vi "Host - REF - MAIN.vi"() -> ()   [LabVIEW 2015]
doc: "This VI initializes de FPGA VI and then configures the DMA FIFO to read streaming data from the FPGA. Once the data is read from the FIFO it is de-interleaved and organized by channels."
uses:
  <vilib>/LabVIEW Targets/FPGA/cRIO/shared/nicrio_ModuleControls/nicrio_cRIO-9234_DataRatesRing2.ctl
  <vilib>/userdefined/High Color/nirio_resource_hc.ctl
  <vilib>/FPGAPlugInAG/cRIO-9112/niLvFpga_Open_cRIO-9112.vi
  <vilib>/rvi/interface/common/dynamic/niFpgaDynamicAddResources.vi
  <vilib>/FPGAPlugInAG/Dynamic/niLvFpga_Reset_Dynamic.vi
  <vilib>/FPGAPlugInAG/Dynamic/niLvFpga_Run_Dynamic.vi
  <vilib>/rvi/errors/niLvFpgaAdjustHostInterfaceError.vi
  <vilib>/rvi/interface/common/niFpgaWaitOnOcc.vi
  <vilib>/RVI Host/nirviSupport.llb/nirviErrorClusterFromErrorCode.vi
  <vilib>/FPGAPlugInAG/Dynamic/niLvFpga_Close_Dynamic.vi
  <vilib>/rvi/interface/nirviOpenFPGA/nirviOpenFPGA.xnode
  FPGA Bitfiles/REF1 - 2 Modules/AmbientSynchrono_FPGATarget2_Target-REF1-mod6-7.lvbitx
  <vilib>/rvi/interface/nirviMethod/nirviMethod.xnode
  <vilib>/rvi/interface/nirviReadWriteControl/nirviReadWriteControl.xnode
  <vilib>/rvi/interface/nirviCloseFPGA/nirviCloseFPGA.xnode
  <vilib>/rvi/interface/Simulation/niFpgaSimulationCallBeginRW.vi
  <vilib>/rvi/errors/niLvFpgaMergeErrorWithErrorCode.vi
  <vilib>/FPGAPlugInAG/Dynamic/niLvFpga_ReadFifo_Dynamic.vi
  NiFpgaLv.dll
  <vilib>/FPGAPlugInAG/Dynamic/niLvFpga_ConfigureFifo_Dynamic.vi
  <vilib>/FPGAPlugInAG/Dynamic/niLvFpga_StartFifo_Dynamic.vi
  <vilib>/rvi/interface/nirviMethod/StockFPGA_InlinedMethodWaitForSingleIRQ.vi
  <vilib>/FPGAPlugInAG/Dynamic/niLvFpga_WaitOnIrq_Dynamic.vi
  <vilib>/FPGAPlugInAG/Dynamic/niLvFpga_AcknowledgeIrq_Dynamic.vi
  <vilib>/FPGAPlugInAG/Dynamic/niLvFpga_StopFifo_Dynamic.vi
panel:
  out "Current Free Space (Mb)":dbl
  out "Low on Free Disk Space":bool
  in  "Save Type":u16(ring) items=["USB", "cRIO"]
  out "?":dbl[][](graph)
  out "Bin Header Check":i32
  in  "Filename":string
  out "UTC offset valid":bool
  out "UTC Offset":i8
  out "Satellites":u8
  out "Antenna Status":T1(ring)
  out "Offset From Time Reference":i32
  out "FPGA Timekeeper locked":bool
  out "GPS status":T2(ring)
  in  "Resource Name":T3 caption="RIO Device"
  out "error out":errorcluster
  out "Elements Remaining":u32
  in  "Stream to Disk":bool
  out "Module Underflow":bool
  out "DMA FIFO Full":bool
  in  "stop":bool
  in  "Data Rate":T4=31 items=["51.200 kS/s (NI 9234)"=1, "25.600 kS/s (NI 9234)"=2, "17.067 kS/s (NI 9234)"=3, "12.800 kS/s (NI 9234)"=4, "10.240 kS/s (NI 9234)"=5, "8.533 kS/s (NI 9234)"=6, "7.314 kS/s (NI 9234)"=7, "6.400 kS/s (NI 9234)"=8, "5.689 kS/s (NI 9234)"=9, "5.120 kS/s (NI 9234)"=10, "4.654 kS/s (NI 9234)"=11, "4.267 kS/s (NI 9234)"=12, "3.938 kS/s (NI 9234)"=13, "3.657 kS/s (NI 9234)"=14, "3.413 kS/s (NI 9234)"=15, "3.200 kS/s (NI 9234)"=16, "3.012 kS/s (NI 9234)"=17, "2.845 kS/s (NI 9234)"=18, "2.695 kS/s (NI 9234)"=19, "2.560 kS/s (NI 9234)"=20, "2.438 kS/s (NI 9234)"=21, "2.328 kS/s (NI 9234)"=22, "2.226 kS/s (NI 9234)"=23, "2.133 kS/s (NI 9234)"=24, "2.048 kS/s (NI 9234)"=25, "1.969 kS/s (NI 9234)"=26, "1.896 kS/s (NI 9234)"=27, "1.829 kS/s (NI 9234)"=28, "1.765 kS/s (NI 9234)"=29, "1.707 kS/s (NI 9234)"=30, "1.652 kS/s (NI 9234)"=31]
  in  "Samples per Channel":u32=3200
  out "RT Buffer Backlog [%]":dbl(slide) scale=0.0..100.0
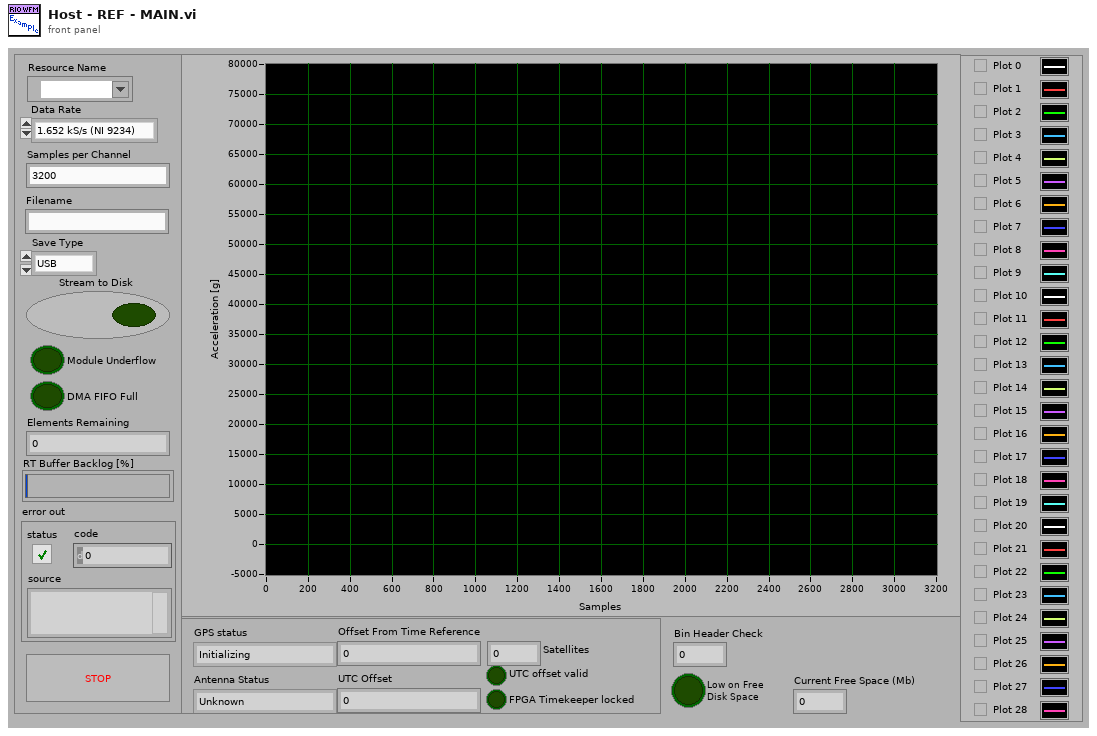
[diagram p1: front panel]
types:
  T1 = enum8{"Unknown", "Normal", "Absent", "Overcurrent"}
  T2 = enum8{"Initializing", "Normal", "Unable to get fix"}
  T3 = typedef "nirio_resource_hc.ctl" = tag
  T4 = typedef "nicrio_cRIO-9234_DataRatesRing2.ctl" = u8
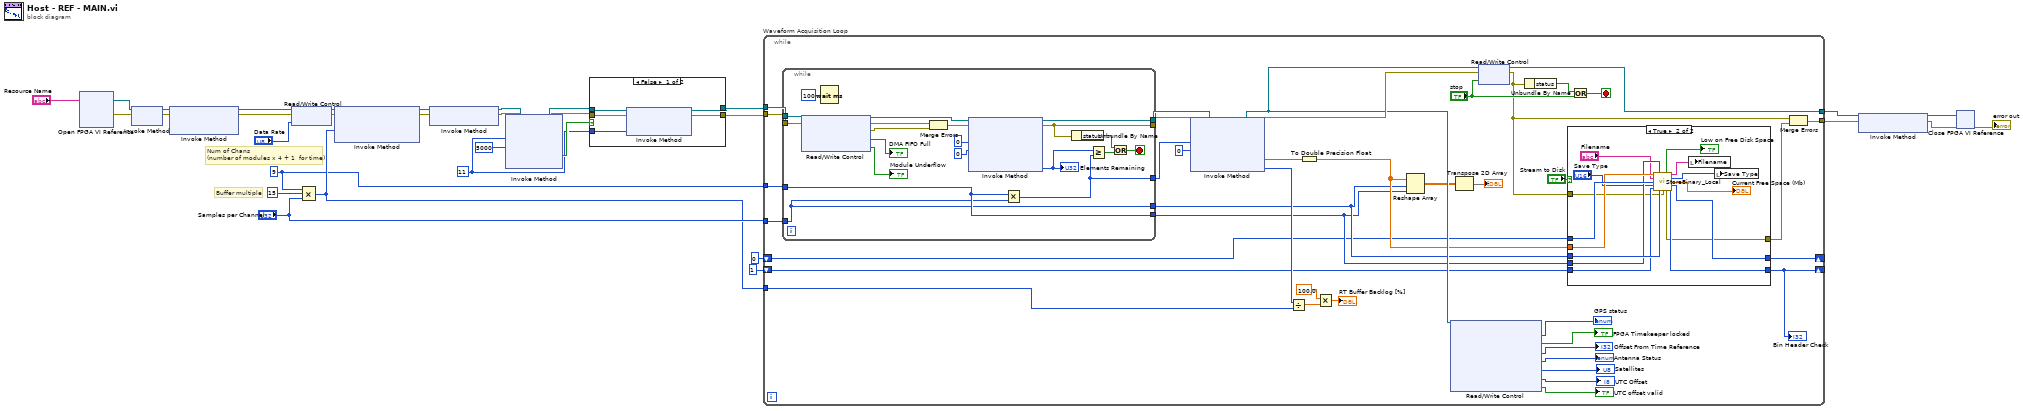
[diagram p0: block diagram]
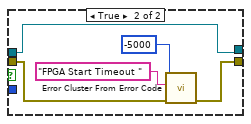
[diagram p2: hidden frame]
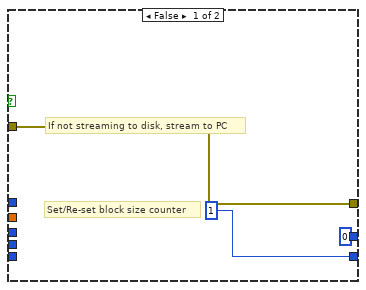
[diagram p3: hidden frame]
diagram:
  w19 = 11 ("IRQ Number(s)")
  w9 = u32 9 ("value")
  # "Buffer multiple"
  # "Num of Chans\n(number of modules x 4 + 1  for time)"
  n1 = xnode "Open FPGA VI Reference"("resource name"="Resource Name") -> ("FPGA VI Reference Out"=w10:refnum<k20>, "error out"=w11:errorcluster)  [unwired: 1 in]
  n2 = xnode "Invoke Method"("FPGA VI Reference In"=w10, "error in"=w11) -> ("FPGA VI Reference Out"=w13:refnum<k20>, "error out"=w12:errorcluster)
  n3 = xnode "Invoke Method"("FPGA VI Reference In"=w13, "error in"=w12) -> ("FPGA VI Reference Out"=w30:refnum<k20>, "error out"=w28:errorcluster)  [unwired: 1 in]
  n4 = xnode "Read/Write Control"("FPGA VI Reference In"=w30, "error in"=w28, "Data Rate"="Data Rate") -> ("FPGA VI Reference Out"=w25:refnum<k20>, "error out"=w24:errorcluster)
  n5 = Compound Arithmetic op=MULTIPLY(w9, u32 15 ("value"), "Samples per Channel") -> (w14:u32)
  n6 = xnode "Invoke Method"("FPGA VI Reference In"=w25, "error in"=w24, "Requested Depth"=w14) -> ("FPGA VI Reference Out"=w26:refnum<k20>, "error out"=w27:errorcluster)  [unwired: 1 out]
  n7 = xnode "Invoke Method"("FPGA VI Reference In"=w26, "error in"=w27) -> ("FPGA VI Reference Out"=w18:refnum<k20>, "error out"=w17:errorcluster)
  n8 = xnode "Invoke Method"("FPGA VI Reference In"=w18, "error in"=w17, "IRQ Number(s)"=w19, "Timeout (ms)"=5000) -> ("FPGA VI Reference Out"=w23:refnum<k20>, "error out"=w22:errorcluster, "Timed Out"=w20:bool)  [unwired: 1 out]
  n9 = case shown="False" w20 {
    tunnel: w23 -> [w37 w39]
    tunnel: w22 -> [w36 w38]
    tunnel: [w35 w39] -> w16
    tunnel: [w34 w40] -> w15
    tunnel: w19 -> [w33 _]
    frame False {
      n10 = xnode "Invoke Method"("FPGA VI Reference In"=w37, "error in"=w36, "IRQ Number(s)"=w33) -> ("FPGA VI Reference Out"=w35:refnum<k20>, "error out"=w34:errorcluster)
    }
    frame True {
      n11 = call <vilib>:"Error Cluster From Error Code.vi"("error in (no error)"=w38, "error message (\"\")"="FPGA Start Timeout " ("error message (\"\")"), "error code (0)"=-5000) -> ("error out"=w40:errorcluster)  [unwired: 1 in, 5 out]
    }
  }
  n12 = while "Waveform Acquisition Loop" {
    tunnel: [w64] -> w6
    tunnel: "Samples per Channel" -> [w73]
    tunnel: w16 -> [w70]
    tunnel: w15 -> [w69]
    tunnel: w14 -> [w75]
    tunnel: [w52] -> w5
    tunnel: w9 -> [w66]
    shift-right: [w50] -> _
    shift-left: 1 -> [w51]
    shift-right: [w44] -> _
    shift-left: u8 0 ("NewFnameCount") -> [w43]
    stop <- w71 stop-if-true
    n13 = while {
      tunnel: [w120] -> w82
      tunnel: [w119] -> w81
      tunnel: [w118] -> w74
      tunnel: w73 -> [w102]
      tunnel: [w103] -> w53
      tunnel: w70 -> [w117]
      tunnel: w69 -> [w116]
      tunnel: [w102] -> w54
      tunnel: w66 -> [w103]
      stop <- w104 stop-if-true
      n14 = xnode "Read/Write Control"("FPGA VI Reference In"=w117, "error in"=w116) -> ("FPGA VI Reference Out"=w115:refnum<k20>, "error out"=w114:errorcluster, "FPGA Error"=w113:errorcluster, "DMA FIFO Full"=→"DMA FIFO Full":bool, "Module Underflow"=→"Module Underflow":bool)
      n15 = Wait (ms)(milliseconds to wait=u32 100) -> ()  [unwired: 1 out]
      n16 = Merge Errors(w114, w113) -> (w112:errorcluster)
      n17 = xnode "Invoke Method"("FPGA VI Reference In"=w115, "error in"=w112, "Number of Elements"=u32 0, "Timeout (ms)"=0) -> ("FPGA VI Reference Out"=w120:refnum<k20>, "error out"=w119:errorcluster, "Elements Remaining"=w107:u32)  [unwired: 1 out]
      "Elements Remaining" <- w107
      n18 = Multiply(x=w103, y=w102) -> (x*y=w118:u32)
      n19 = Unbundle By Name(w119) -> ("status"=w105:bool)
      n20 = Greater Or Equal?(x=w107, y=w118) -> (x >= y?=w106:bool)
      n21 = Or(x=w105, y=w106) -> (x .or. y?=w104:bool)
    }
    n22 = xnode "Invoke Method"("FPGA VI Reference In"=w82, "error in"=w81, "Number of Elements"=w74, "Timeout (ms)"=0) -> ("FPGA VI Reference Out"=w63:refnum<k20>, "error out"=w68:errorcluster, "Data"=w46:fxp<+/-,64,44>[], "Elements Remaining"=w76:u32)
    n23 = Divide(x=w76, y=w75) -> (x/y=w79:dbl)
    n24 = To Double Precision Float(number=w46) -> (double precision float=w55:dbl[])
    n25 = Multiply(x=100.0, y=w79) -> (x*y=→"RT Buffer Backlog [%]":dbl)
    n26 = Reshape Array(w55, w54, w53) -> (w48:dbl[][])
    n27 = xnode "Read/Write Control"("FPGA VI Reference In"=w63) -> ("GPS status"=→"GPS status":T2, "FPGA Timekeeper locked"=→"FPGA Timekeeper locked":bool, "offset from time reference"=→"Offset From Time Reference":i32, "antenna status"=→"Antenna Status":T1, "satellites available"=→"Satellites":u8, "UTC offset"=→"UTC Offset":i8, "UTC offset valid"=→"UTC offset valid":bool)  [unwired: 1 in, 2 out]
    n28 = Transpose 2D Array(2D array=w48) -> (transposed array=→"?":dbl[][])
    n29 = xnode "Read/Write Control"("FPGA VI Reference In"=w63, "error in"=w68, "Stop"="stop") -> ("FPGA VI Reference Out"=w64:refnum<k20>, "error out"=w49:errorcluster)
    n30 = Unbundle By Name(w49) -> ("status"=w72:bool)
    n31 = case shown="True" "Stream to Disk" {
      tunnel: w55 -> [_ w99]
      tunnel: w54 -> [_ w98]
      tunnel: w53 -> [_ w97]
      tunnel: w51 -> [_ w96]
      tunnel: [1 w88] -> w50
      tunnel: w49 -> [w85 w87]
      tunnel: [w85 w86] -> w45
      tunnel: w43 -> [_ w100]
      tunnel: [u8 0 ("NewFnameCount") w90] -> w44
      frame False {
        # "Set/Re-set block size counter"
        # "If not streaming to disk, stream to PC"
      }
      frame True {
        n32 = call "StoreBinary_Local.vi"("Data Array"=w99, "Number of Channels"=w97, "Filename"="Filename", "Fname Increment"=w100, "Save Type"="Save Type", "Bin Header"=w96, "Block Size"=w98, "error in (no error)"=w87) -> ("Low on Free Disk Space"=→"Low on Free Disk Space":bool, "New Fname"=w92:string, "New Save Type"=w91:u16, "Current Free Space (Mb)"=→"Current Free Space (Mb)":dbl, "NewFnameCount"=w90:u8, "error out"=w86:errorcluster, "Counter Out"=w88:i32)  [unwired: 1 in]
        n33 = local write "Filename"(w92) -> ()
        n34 = local write "Save Type"(w91) -> ()
      }
    }
    "Bin Header Check" <- w50
    n35 = Or(x=w72, y="stop") -> (x .or. y?=w71:bool)
    n36 = Merge Errors(w49, w45) -> (w52:errorcluster)
  }
  n37 = xnode "Invoke Method"("FPGA VI Reference In"=w6, "error in"=w5) -> ("FPGA VI Reference Out"=w3:refnum<k20>, "error out"=w2:errorcluster)
  n38 = xnode "Close FPGA VI Reference"("FPGA VI Reference In"=w3, "error in"=w2) -> ("error out"=→"error out":errorcluster)
